vi "parseStepMotorError.vi"(8 "error in (no error)":errorcluster, 10 "DynamicFrameParser":refnum<class "DynamicFrameParser.lvclass">, 11 "HardPointActuator in":refnum<class "HPILC.lvclass">) -> (0 "error out":errorcluster, 3 "HardPointActuator out":refnum<class "HPILC.lvclass">)   [LabVIEW 2015, in "RTHPILC.lvlib" / "HPILC.lvclass"]
uses:
  HPILC.lvclass
  Common_RT_Modbus/DynamicFrameParser/DynamicFrameParser.lvclass
  HPILC.lvclass/HPILC.ctl
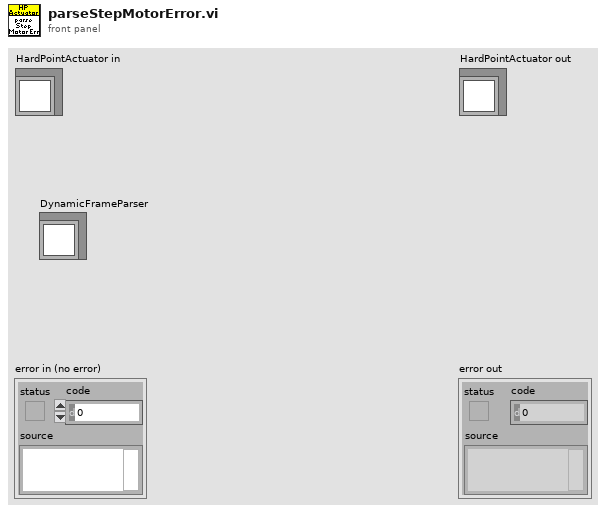
[diagram p1: front panel]
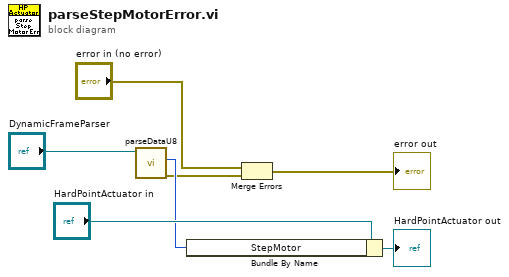
[diagram p0: block diagram]
diagram:
  n1 = call "parseDataU8.vi"("FrameParser in"="DynamicFrameParser") -> ("error out"=w1:errorcluster, "Data"=w2:u8)  [unwired: 8 in, 1 out]
  n2 = Bundle By Name(cluster="HardPointActuator in", "StepMotor"=w2) -> (→"HardPointActuator out":refnum<class "HPILC.lvclass">)
  n3 = Merge Errors("error in (no error)", w1) -> (→"error out":errorcluster)
